vi "Write Vpmt.vi"(8 "error in (no error)":errorcluster, 10 "Vpmt":dbl[](array[numeric]), 11 "Update PMT Gains MSG in":refnum<class "Update PMT Gains MSG.lvclass">) -> (0 "error out":errorcluster, 3 "Update PMT Gains MSG out":refnum<class "Update PMT Gains MSG.lvclass">)   [LabVIEW 2014, in "eCRDS Library.lvlib" / "Update PMT Gains MSG.lvclass"]
uses:
  Update PMT Gains MSG.lvclass
  Update PMT Gains MSG.lvclass/Update PMT Gains MSG.ctl
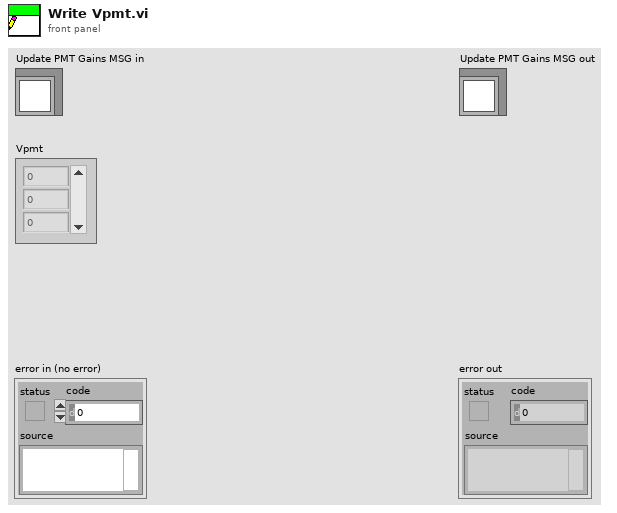
[diagram p1: front panel]
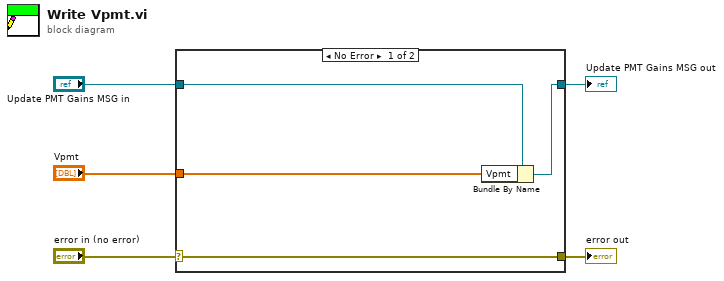
[diagram p0: block diagram]
diagram:
  n1 = case shown="No Error" "error in (no error)" {
    selector: "error in (no error)" -> [w9 w10]
    tunnel: [w9 w10] -> w4
    tunnel: [w7 w11] -> w2
    tunnel: "Update PMT Gains MSG in" -> [w8 w11]
    tunnel: "Vpmt" -> [w6 _]
    frame No Error {
      n2 = Bundle By Name(cluster=w8, "Vpmt"=w6) -> (w7:refnum<class "Update PMT Gains MSG.lvclass">)
    }
    frame Error {
    }
  }
  "error out" <- w4
  "Update PMT Gains MSG out" <- w2
